vi "Write Particle.vi"(8 "error in (no error)":errorcluster, 10 "Particles":refnum<class "Particle Properties.lvclass">, 11 "DMA in":refnum<class "DMA.lvclass">) -> (0 "error out":errorcluster, 3 "DMA out":refnum<class "DMA.lvclass">)   [LabVIEW 2015, in "DMA.lvclass"]
uses:
  DMA.lvclass
  Particle Class/Particle Properties.lvclass
  DMA.lvclass/DMA.ctl
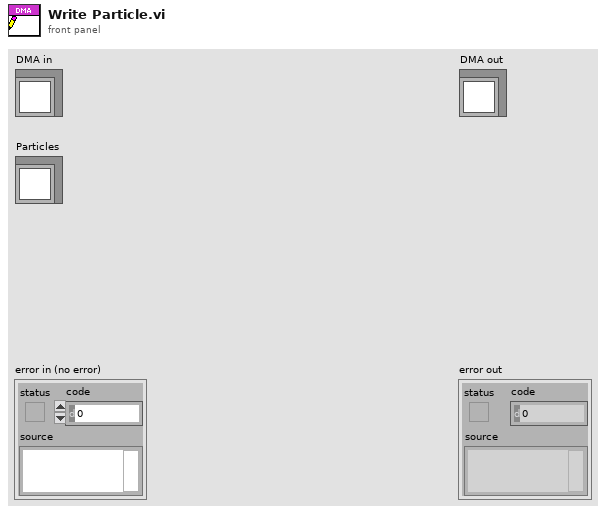
[diagram p1: front panel]
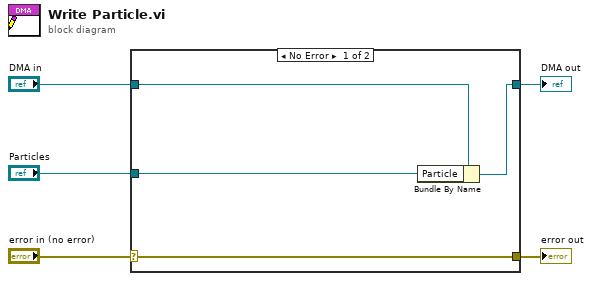
[diagram p0: block diagram]
diagram:
  n1 = case shown="No Error" "error in (no error)" {
    selector: "error in (no error)" -> [w9 w10]
    tunnel: [w9 w10] -> w4
    tunnel: [w7 w11] -> w2
    tunnel: "DMA in" -> [w8 w11]
    tunnel: "Particles" -> [w6 _]
    frame No Error {
      n2 = Bundle By Name(cluster=w8, "Particle"=w6) -> (w7:refnum<class "DMA.lvclass">)
    }
    frame Error {
    }
  }
  "error out" <- w4
  "DMA out" <- w2
